vi "CreatePrivateEvents.vi"(8 "error in (no error)":errorcluster, 11 "SMO.UI":refnum<class "SMO.UI.lvclass">) -> (0 "error out":errorcluster, 3 "SMO.UI out":refnum<class "SMO.UI.lvclass">)   [LabVIEW 2021, in "smo.lvlib" / "SMO.UI.lvclass"]
uses:
  SMO.UI.lvclass
  SMO.UI.lvclass/SMO.UI.ctl
  SMO/SMO.lvclass
panel:
  # "For instructions on how to use the JKI State Machine Objects, examples and video tutorials, visit:\nhttp://jki.net/state-machine-objects/\n\nJKI State Machine Objects™\nhttp://jki.net/state-machine-objects/\nCopyright (C) 2005-2015, JKI <info@jki.net>\nALL RIGHTS RESERVED"
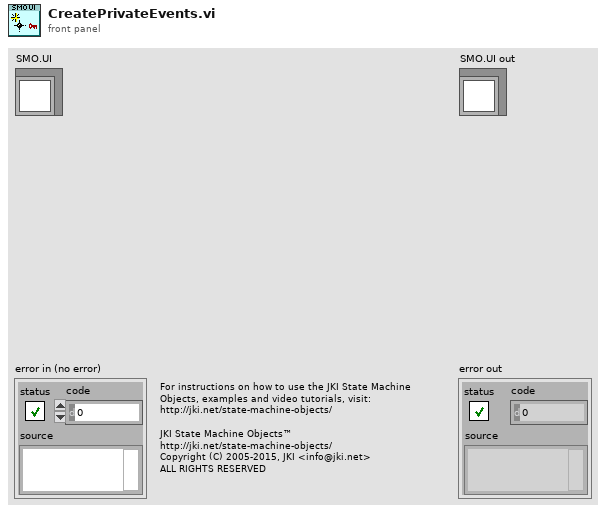
[diagram p1: front panel]
types:
  T1 = typedef "smo.lvlib/SMO.UI.lvclass/PrivateData--Ref.ctl" = refnum<data-value>
  T2 = typedef "smo.lvlib/SMO.UI.lvclass/PrivateData--Cluster.ctl" = cluster{"Public Events":T3, "Private Events":T4}
  T3 = typedef "smo.lvlib/SMO.UI.lvclass/PublicEvents--Cluster.ctl" = cluster{"UI Hidden":refnum<user-event>, "UI State":refnum<user-event>}
  T4 = typedef "smo.lvlib/SMO.UI.lvclass/PrivateEvents--Cluster.ctl" = cluster{"Show-Hide UI":refnum<user-event>}
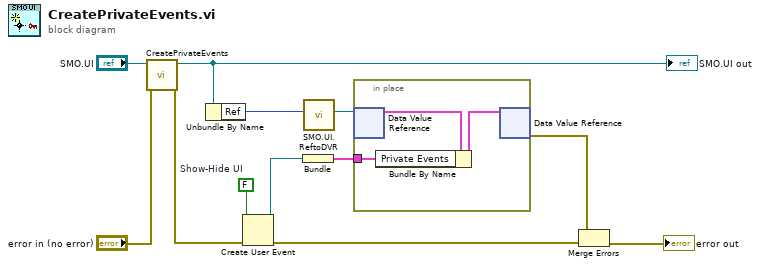
[diagram p0: block diagram]
diagram:
  w5 = FALSE  # Show-Hide UI
  n1 = call-parent "CreatePrivateEvents.vi"("error in (no error)"="error in (no error)", "SMO"="SMO.UI") -> ("error out"=w12:errorcluster, "SMO out"=w1:refnum<class "SMO.UI.lvclass">)  [unwired: 8 in]
  "SMO.UI out" <- w1
  n2 = Unbundle By Name(w1) -> ("Ref"=w7:u32)
  n3 = Create User Event(user event datatype=w5, error in=w12) -> (user event=w3:refnum<user-event>, error out=w10:errorcluster)
  n4 = Bundle("Show-Hide UI"=w3) -> (w4:cluster{"Show-Hide UI":refnum<user-event>})  [unwired: 1 in]
  n5 = call "SMO.UI.ReftoDVR.vi"("Ref"=w7) -> ("Ref"=w6:T1)  [unwired: 10 in]
  n6 = in-place {
    in-place-border: w4 -> [w13]
    n7 = in-place-dvr #1(w6) -> (w15:T2)  [unwired: 1 out]
    n8 = Bundle By Name(cluster=w15, "Private Events"=w13) -> (w14:T2)
    n9 = in-place-dvr #1(w14) -> (w9:errorcluster)  [unwired: 1 out]
  }
  n10 = Merge Errors(w9, w10) -> (→"error out":errorcluster)
